vi "H2Purifier_01.vi"() -> ()   [LabVIEW 2011]
panel:
  in  "MANIFOLD N2":bool
  in  "MANIFOLD H2":bool
  out "String":string
  out "Bleed gas valve":string
  out "UPH Flow valve":string
  in  "Close":bool
  out "Close LED":bool caption="Open"
  in  "Open":bool
  out "Open LED":bool caption="Open"
  in  "Vac\nExhuast":bool
  in  "Step":i16
  in  "OK Button":bool
  out "Feed":bool
  out "Pump":bool
  out "Purge":bool
  out "Evac":bool
  out "H2 (sccm)":dbl
  out "N2 (sccm)":dbl
  in  "Tab Control":enum32{"Start up", "Idle"}(tab)
  # "setpoint to ~100 sccm"
  # "sepoint ~200 sccm\nFlow will drop to ~0 sccm"
  # "H2 Purifier"
  # "AdapTorr"
  # "BLEED\nGAS"
  # "UPH FLOW"
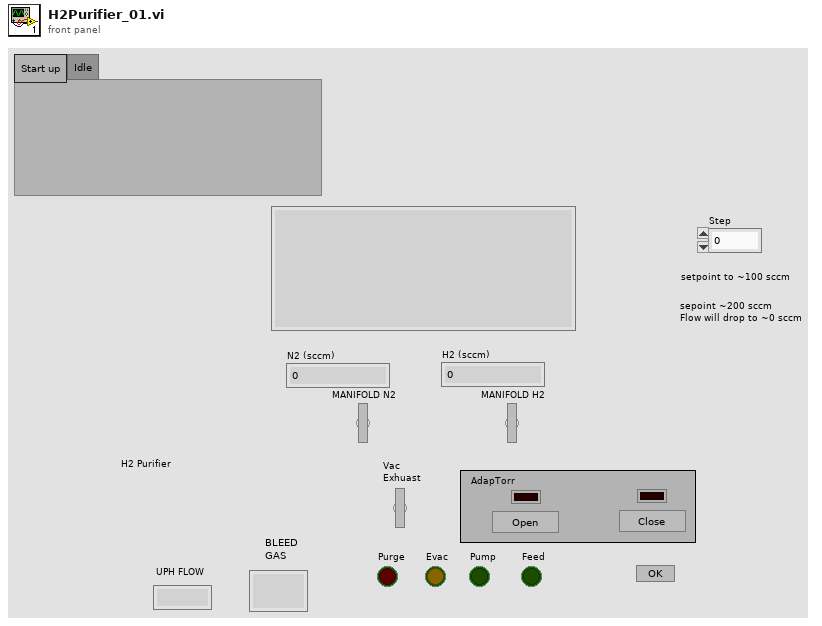
[diagram p1: front panel]
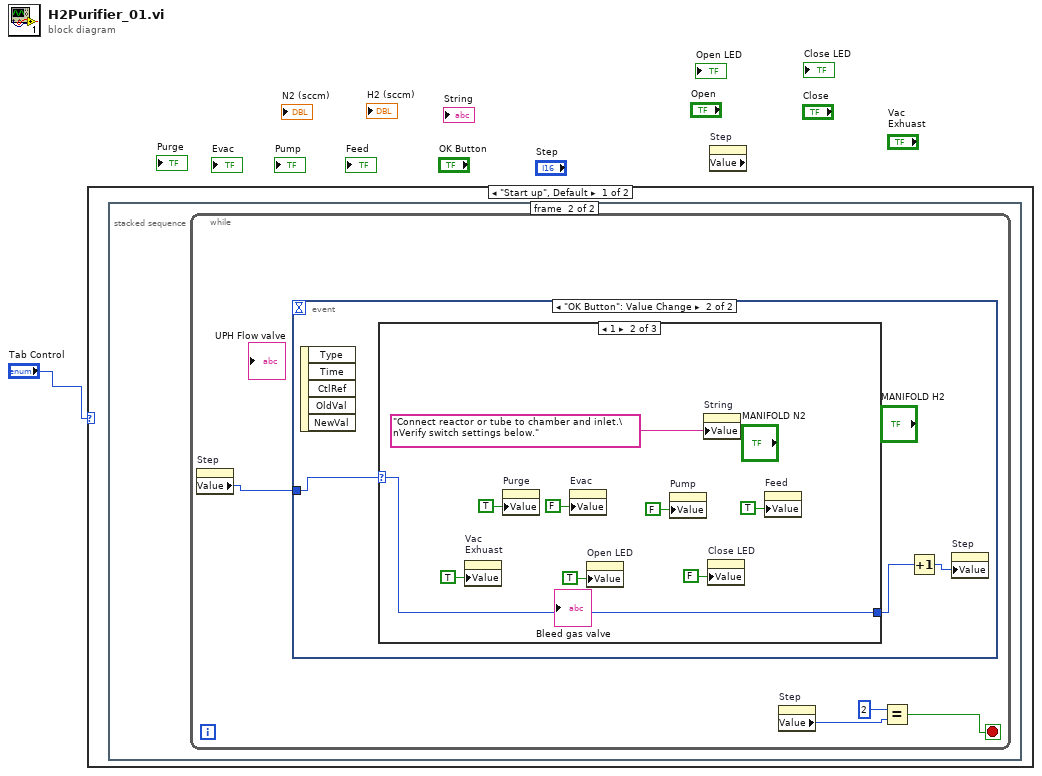
[diagram p0: block diagram]
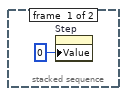
[diagram p2: hidden frame]
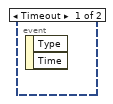
[diagram p3: hidden frame]
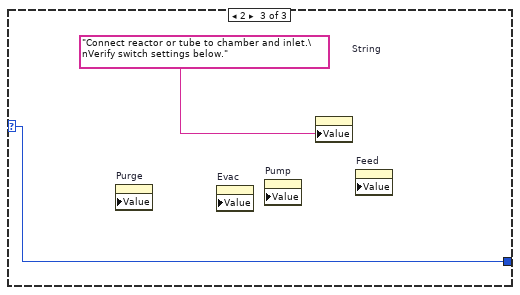
[diagram p5: hidden frame]
diagram:
  n1 = case shown="\"Start up\", Default" "Tab Control" {
    frame "Start up", Default {
      n2 = stacked-sequence {
        frame #0 {
          n3 = property on="Step" class="DigNum (strict)"("Value"=i16 0 ("Step")) -> ()  [unwired: 2 in, 2 out]
        }
        frame #1 {
          n4 = while {
            stop <- w4 stop-if-true
            n5 = property on="Step" class="DigNum (strict)"() -> ("Value"=w3:i16)  [unwired: 2 in, 2 out]
            n6 = event shown="[1] \"OK Button\": Value Change" {
              selector: _ -> [_ _]
              dyn-events: _ -> [_ _]
              timeout: _ -> [_ _]
              tunnel: w3 -> [_ w9]
              event Timeout {
                n7 = event-data() -> ()  [unwired: 1 in, 2 out]
              }
              event "OK Button": Value Change {
                n8 = event-data() -> ()  [unwired: 1 in, 5 out]
                n9 = case shown="1" w9 {
                  selector: w9 -> [w10 w14 w20]
                  tunnel: [w10 w14 w20] -> w7
                  frame 0, Default {
                  }
                  frame 1 {
                    n10 = property on="Vac\nExhuast" class="Bool (strict)"("Value"=TRUE ("Vac\nExhuast")) -> ()  [unwired: 2 in, 2 out]
                    n11 = property on="Purge" class="Bool (strict)"("Value"=TRUE ("Purge")) -> ()  [unwired: 2 in, 2 out]
                    n12 = property on="Evac" class="Bool (strict)"("Value"=FALSE ("Evac")) -> ()  [unwired: 2 in, 2 out]
                    n13 = property on="Open LED" class="Bool (strict)"("Value"=TRUE ("Open LED")) -> ()  [unwired: 2 in, 2 out]
                    n14 = property on="Pump" class="Bool (strict)"("Value"=FALSE ("Pump")) -> ()  [unwired: 2 in, 2 out]
                    n15 = property on="String" class="Str"("Value"="Connect reactor or tube to chamber and inlet.\nVerify switch settings below." ("String")) -> ()  [unwired: 2 in, 2 out]
                    n16 = property on="Close LED" class="Bool (strict)"("Value"=FALSE ("Close LED")) -> ()  [unwired: 2 in, 2 out]
                    n17 = property on="Feed" class="Bool (strict)"("Value"=TRUE ("Feed")) -> ()  [unwired: 2 in, 2 out]
                  }
                  frame 2 {
                    n18 = property on="Purge" class="Bool (strict)" props=["Value"]() -> ()  [unwired: 3 in, 2 out]
                    n19 = property on="Evac" class="Bool (strict)" props=["Value"]() -> ()  [unwired: 3 in, 2 out]
                    n20 = property on="Pump" class="Bool (strict)" props=["Value"]() -> ()  [unwired: 3 in, 2 out]
                    n21 = property on="String" class="Str"("Value"="Connect reactor or tube to chamber and inlet.\nVerify switch settings below." ("String")) -> ()  [unwired: 2 in, 2 out]
                    n22 = property on="Feed" class="Bool (strict)" props=["Value"]() -> ()  [unwired: 3 in, 2 out]
                  }
                }
                n23 = Increment(x=w7) -> (x+1=w8:i16)
                n24 = property on="Step" class="DigNum (strict)"("Value"=w8) -> ()  [unwired: 2 in, 2 out]
              }
            }
            n25 = property on="Step" class="DigNum (strict)"() -> ("Value"=w6:i16)  [unwired: 2 in, 2 out]
            n26 = Equal?(x=i16 2, y=w6) -> (x = y?=w4:bool)
          }
        }
      }
    }
    frame "Idle" {
      n27 = stacked-sequence {
        frame #0 {
        }
      }
    }
  }
  n28 = property on="Step" class="DigNum (strict)" props=["Value"]() -> ()  [unwired: 2 in, 3 out]
